vi "Modify Or Add Variant Attribute.vi"(6 "Initial Value For New Attributes":T1, 8 "error in (no error)":errorcluster, 9 "Increment":T1, 10 "Attribute Name":string, 11 "Variant in":variant) -> (0 "error out":errorcluster, 1 "Modified Attribute Value":T1, 3 "Variant out":variant)   [LabVIEW 2023]
doc: "This VI adds a variant attribute if it does not already exist or modifies an existing attribute without making excessive data copies while accessing the attribute data."
uses:
  Lookup Table Data.ctl
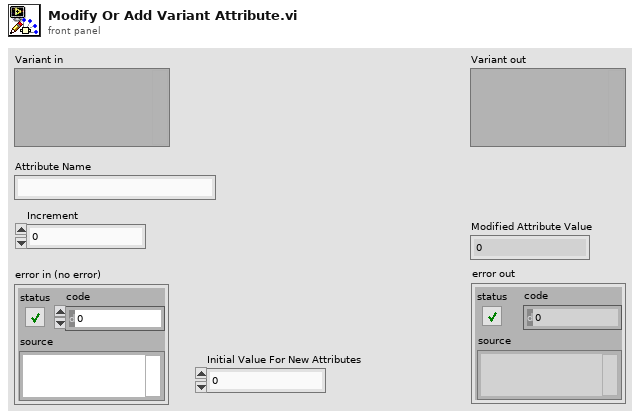
[diagram p1: front panel]
types:
  T1 = typedef "Lookup Table Data.ctl" = u32
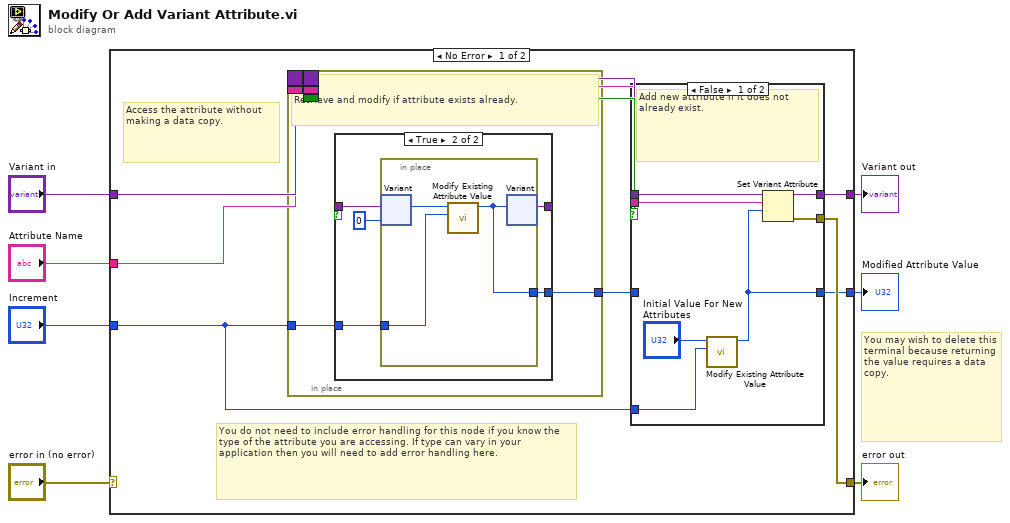
[diagram p0: block diagram]
diagram:
  # "You may wish to delete this terminal because returning the value requires a data copy."
  n1 = case shown="No Error" "error in (no error)" {
    selector: "error in (no error)" -> [_ w41]
    tunnel: "Variant in" -> [w17 w42]
    tunnel: "Attribute Name" -> [w16 _]
    tunnel: "Increment" -> [w12 _]
    tunnel: [w11 w42] -> w4
    tunnel: [w10 w41] -> w2
    tunnel: [w8 _] -> w1
    frame No Error {
      # "Access the attribute without making a data copy."
      # "You do not need to include error handling for this node if you know the type of the attribute you are accessing. If type can vary in your application then you will need to add error handling here."
      n2 = in-place {
        border: w17 -> [_]
        border: w16 -> [_]
        border: [_] -> w14
        border: [_] -> w13
        border: [_] -> w15
        in-place-border: w12 -> [w19]
        in-place-border: [w18] -> w9
        # "Retrieve and modify if attribute exists already."
        n3 = case shown="True" w22 {
          tunnel: w20 -> [w23 w28]
          tunnel: [w23 w25] -> w21
          tunnel: w19 -> [_ w26]
          tunnel: [_ w24] -> w18
          frame False {
          }
          frame True {
            n4 = in-place {
              in-place-border: w26 -> [w30]
              in-place-border: [w29] -> w24
              n5 = in-place-variant #1(w28, T1 0 ("Increment")) -> (w31:T1)  [unwired: 1 out]
              n6 = call "Modify Existing Attribute Value.vi"("Increment"=w30, "Value in"=w31) -> ("Value out"=w29:T1)  [unwired: 9 in]
              n7 = in-place-variant #1(w29) -> (w25:variant)  [unwired: 1 out]
            }
          }
        }
      }
      n8 = case shown="False" w15 {
        tunnel: w14 -> [w38 w40]
        tunnel: w13 -> [w37 _]
        tunnel: w12 -> [w33 _]
        tunnel: [w36 w40] -> w11
        tunnel: [w35 _] -> w10
        tunnel: w9 -> [_ w39]
        tunnel: [w32 w39] -> w8
        frame False {
          # "Add new attribute if it does not already exist."
          n9 = call "Modify Existing Attribute Value.vi"("Increment"=w33, "Value in"="Initial Value For New Attributes") -> ("Value out"=w32:T1)  [unwired: 9 in]
          n10 = Set Variant Attribute(Variant=w38, name=w37, value=w32) -> (Variant out=w36:variant, error out=w35:errorcluster)  [unwired: 1 in, 1 out]
        }
        frame True {
        }
      }
    }
    frame Error {
    }
  }
  "Variant out" <- w4
  "error out" <- w2
  "Modified Attribute Value" <- w1
